vi "Numero de espaçadores.vi"(8 "error in (no error)":errorcluster, 11 "Dados SP":T1={"Condutor"={"Pc (N/m)"=0.0, "Mod.Young (N/m²)"=0.0, "Dil.Term.c (m/°C)"=0.0, "Área  (m²)"=0.0, "Tração EDS (N)"=0.0, "Tração Torig(N)"=0.0, "Tração Talta (N)"=0.0}, "Suporte"={"Ps (N/m)"=0.0, "Es (N/m²)"=0.0, "DTc (1/°C)"=0.0, "Área sup (m²)"=0.0, "Tração EDS sup (N)"=0.0, "Tração AT sup (N)"=0.0, "Flecha sup AT (m)"=0.0}, "Projeto"={"Temp. EDS (°C)"=0.0, "Lim.original (°C)"=0.0, "Lim.extend. (°C)"=0.0, "N. cabo/fase"=1.0}, "Vetor de dados"={"Coor.X.esp"=[], "Coor.Y.Esp."=[], "Sub.vao X"=[], "Sub.vao Y"=[], "CoordY.sup"=[], "CoordX.sup"=[]}, "Subvão"={"N. Esp."=0.0, "F.lim (m)"=0.0, "Ext.calc"=0.0, "Ext.definido"=0.0, "Comp.cabo"=0.0, "Ext.55%"=0.0, "Tração sub\nAT (N)"=0.0, "Ext.sel."=0.0, "Flecha lim.\ncalc (m)"=0.0}, "Vão"={"Extensão (m)"=0.0, "Desnivel (m)"=0.0, "Ext.Lim sub (m)"=0.0, "Flecha à 60 °C"=0.0}} {"Projeto"."N. cabo/fase" min=1.0 max=8.0 step=1.0 format="%#_1f"}) -> (0 "error out":errorcluster, 3 "Dados SP Out":T1={"Condutor"={"Pc (N/m)"=0.0, "Mod.Young (N/m²)"=0.0, "Dil.Term.c (m/°C)"=0.0, "Área  (m²)"=0.0, "Tração EDS (N)"=0.0, "Tração Torig(N)"=0.0, "Tração Talta (N)"=0.0}, "Suporte"={"Ps (N/m)"=0.0, "Es (N/m²)"=0.0, "DTc (1/°C)"=0.0, "Área sup (m²)"=0.0, "Tração EDS sup (N)"=0.0, "Tração AT sup (N)"=0.0, "Flecha sup AT (m)"=0.0}, "Projeto"={"Temp. EDS (°C)"=0.0, "Lim.original (°C)"=0.0, "Lim.extend. (°C)"=0.0, "N. cabo/fase"=1.0}, "Vetor de dados"={"Coor.X.esp"=[], "Coor.Y.Esp."=[], "Sub.vao X"=[], "Sub.vao Y"=[], "CoordY.sup"=[], "CoordX.sup"=[]}, "Subvão"={"N. Esp."=0.0, "F.lim (m)"=0.0, "Ext.calc"=0.0, "Ext.definido"=0.0, "Comp.cabo"=0.0, "Ext.55%"=0.0, "Tração sub\nAT (N)"=0.0, "Ext.sel."=0.0, "Flecha lim.\ncalc (m)"=0.0}, "Vão"={"Extensão (m)"=0.0, "Desnivel (m)"=0.0, "Ext.Lim sub (m)"=0.0, "Flecha à 60 °C"=0.0}} {"Projeto"."N. cabo/fase" min=1.0 max=8.0 step=1.0 format="%#_1f"})   [LabVIEW 2020]
uses:
  controles/SP data.ctl
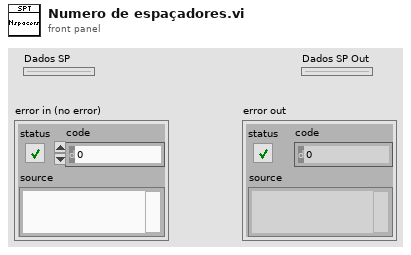
[diagram p1: front panel]
types:
  T1 = typedef "SP data.ctl" = cluster{"Condutor":cluster{"Pc (N/m)":dbl, "Mod.Young (N/m²)":dbl, "Dil.Term.c (m/°C)":dbl, "Área  (m²)":dbl, "Tração EDS (N)":dbl, "Tração Torig(N)":dbl, "Tração Talta (N)":dbl}, "Suporte":cluster{"Ps (N/m)":dbl, "Es (N/m²)":dbl, "DTc (1/°C)":dbl, "Área sup (m²)":dbl, "Tração EDS sup (N)":dbl, "Tração AT sup (N)":dbl, "Flecha sup AT (m)":dbl}, "Projeto":cluster{"Temp. EDS (°C)":dbl, "Lim.original (°C)":dbl, "Lim.extend. (°C)":dbl, "N. cabo/fase":dbl}, "Vetor de dados":cluster{"Coor.X.esp":dbl[], "Coor.Y.Esp.":dbl[], "Sub.vao X":dbl[], "Sub.vao Y":dbl[], "CoordY.sup":dbl[], "CoordX.sup":dbl[]}, "Subvão":cluster{"N. Esp.":dbl, "F.lim (m)":dbl, "Ext.calc":dbl, "Ext.definido":dbl, "Comp.cabo":dbl, "Ext.55%":dbl, "Tração sub\nAT (N)":dbl, "Ext.sel.":dbl, "Flecha lim.\ncalc (m)":dbl}, "Vão":cluster{"Extensão (m)":dbl, "Desnivel (m)":dbl, "Ext.Lim sub (m)":dbl, "Flecha à 60 °C":dbl}}
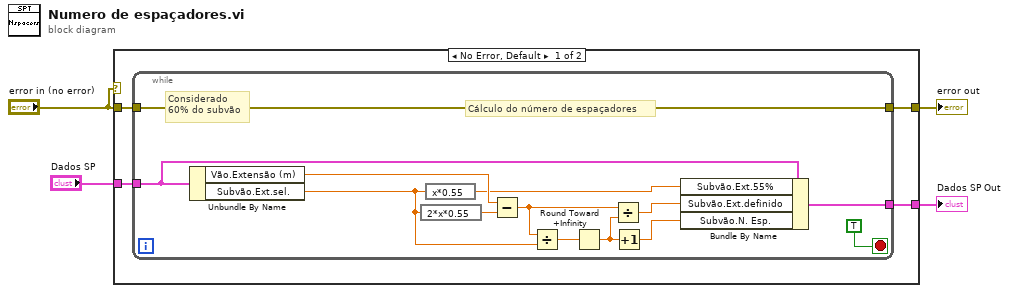
[diagram p0: block diagram]
diagram:
  n1 = case shown="No Error, Default" "error in (no error)" {
    tunnel: "Dados SP" -> [w8 w22]
    tunnel: "error in (no error)" -> [w7 w23]
    tunnel: [w6 w23] -> w3
    tunnel: [w5 w22] -> w2
    frame No Error {
      n2 = while {
        tunnel: w8 -> [w14]
        tunnel: w7 -> [w16]
        tunnel: [w16] -> w6
        tunnel: [w12] -> w5
        stop <- TRUE stop-if-true
        # "Considerado \n60% do subvão"
        # "Cálculo do número de espaçadores"
        n3 = Unbundle By Name(w14) -> ("Vão.Extensão (m)"=w18:dbl, "Subvão.Ext.sel."=w15:dbl)
        n4 = expression code="2*x*0.55"(w15) -> (w19:dbl)
        n5 = expression code="x*0.55"(w15) -> (w13:dbl)
        n6 = Subtract(x=w18, y=w19) -> (x-y=w21:dbl)
        n7 = Divide(x=w21, y=w15) -> (x/y=w20:dbl)
        n8 = Round Toward +Infinity(x=w20) -> (ceil(x): smallest int >= x=w10:dbl)
        n9 = Divide(x=w21, y=w10) -> (x/y=w11:dbl)
        n10 = Increment(x=w10) -> (x+1=w9:dbl)
        n11 = Bundle By Name(cluster=w14, "Subvão.Ext.55%"=w13, "Subvão.Ext.definido"=w11, "Subvão.N. Esp."=w9) -> (w12:T1)
      }
    }
    frame Error {
    }
  }
  "Dados SP Out" <- w2
  "error out" <- w3
